vi "Limelight_Differential.vi"() -> (0 "DriveCommand":dbl(knob)=-0.0 scale=-1.0..1.0, 1 "SteerCommand":dbl(knob)=nan scale=-1.0..1.0, 3 "TargetValid":bool)   [LabVIEW 2020]
uses:
  Robot Global Data.vi
panel:
  out "Copy of DriveCommand":dbl format="%_6g"
  out "Limelight tv":dbl
  out "Limelight ta":dbl
  out "Limelight tx":dbl
  out "MaxDrive":dbl(slide)=0.6824817518248175 min=0.0 max=1.0 step=0.01 scale=0.0..1.0
  out "DriveK":dbl(slide)=0.26277372262773724 min=0.0 max=1.0 step=0.05 scale=0.0..1.0
  out "Limelight Goal Area":dbl(slide)=14.872262773722628 min=0.1 max=25.0 step=0.25 scale=0.0..25.0
  out "AimDeadband":dbl min=0.0 max=10.0 step=0.25
  out "MinSteerCommand":dbl(slide)=0.2717391304347826 min=0.0 max=0.5 step=0.05 scale=0.0..0.5
  out "SteeringK":dbl(slide)=0.025362318840579712 min=0.0 max=0.25 step=0.01 scale=0.0..0.25
  # "// These numbers must be tuned for your Robot!  Be careful!\n\n final double STEER_K = 0.03;                    \n// how hard to turn toward the target\n\n\n\n\n \n\nfinal double DESIRED_TARGET_AREA = 13.0;        \n// Area of the target when the robot reaches the wall\n\n\n\nfinal double DRIVE_K = 0.26;                   \n // how hard to drive fwd toward the target\n\n \n \nfinal double MAX_DRIVE = 0.7;                   \n// Simple speed limit so we don't drive too fast"
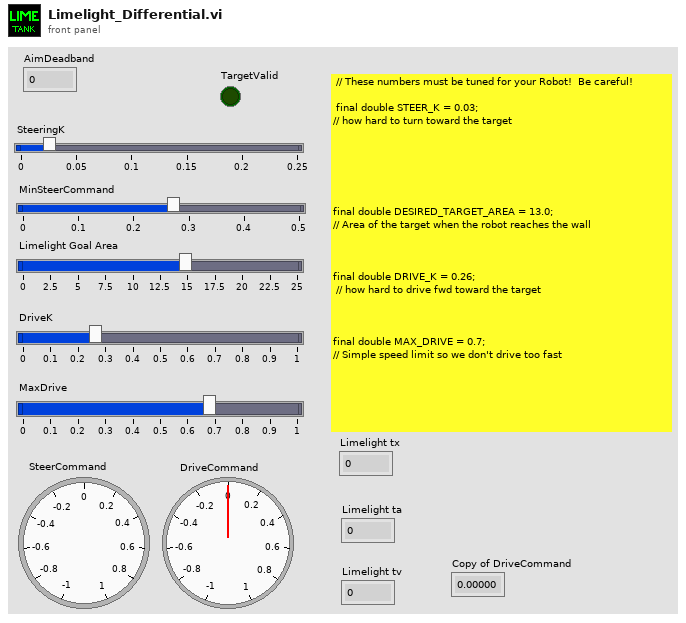
[diagram p1: front panel]
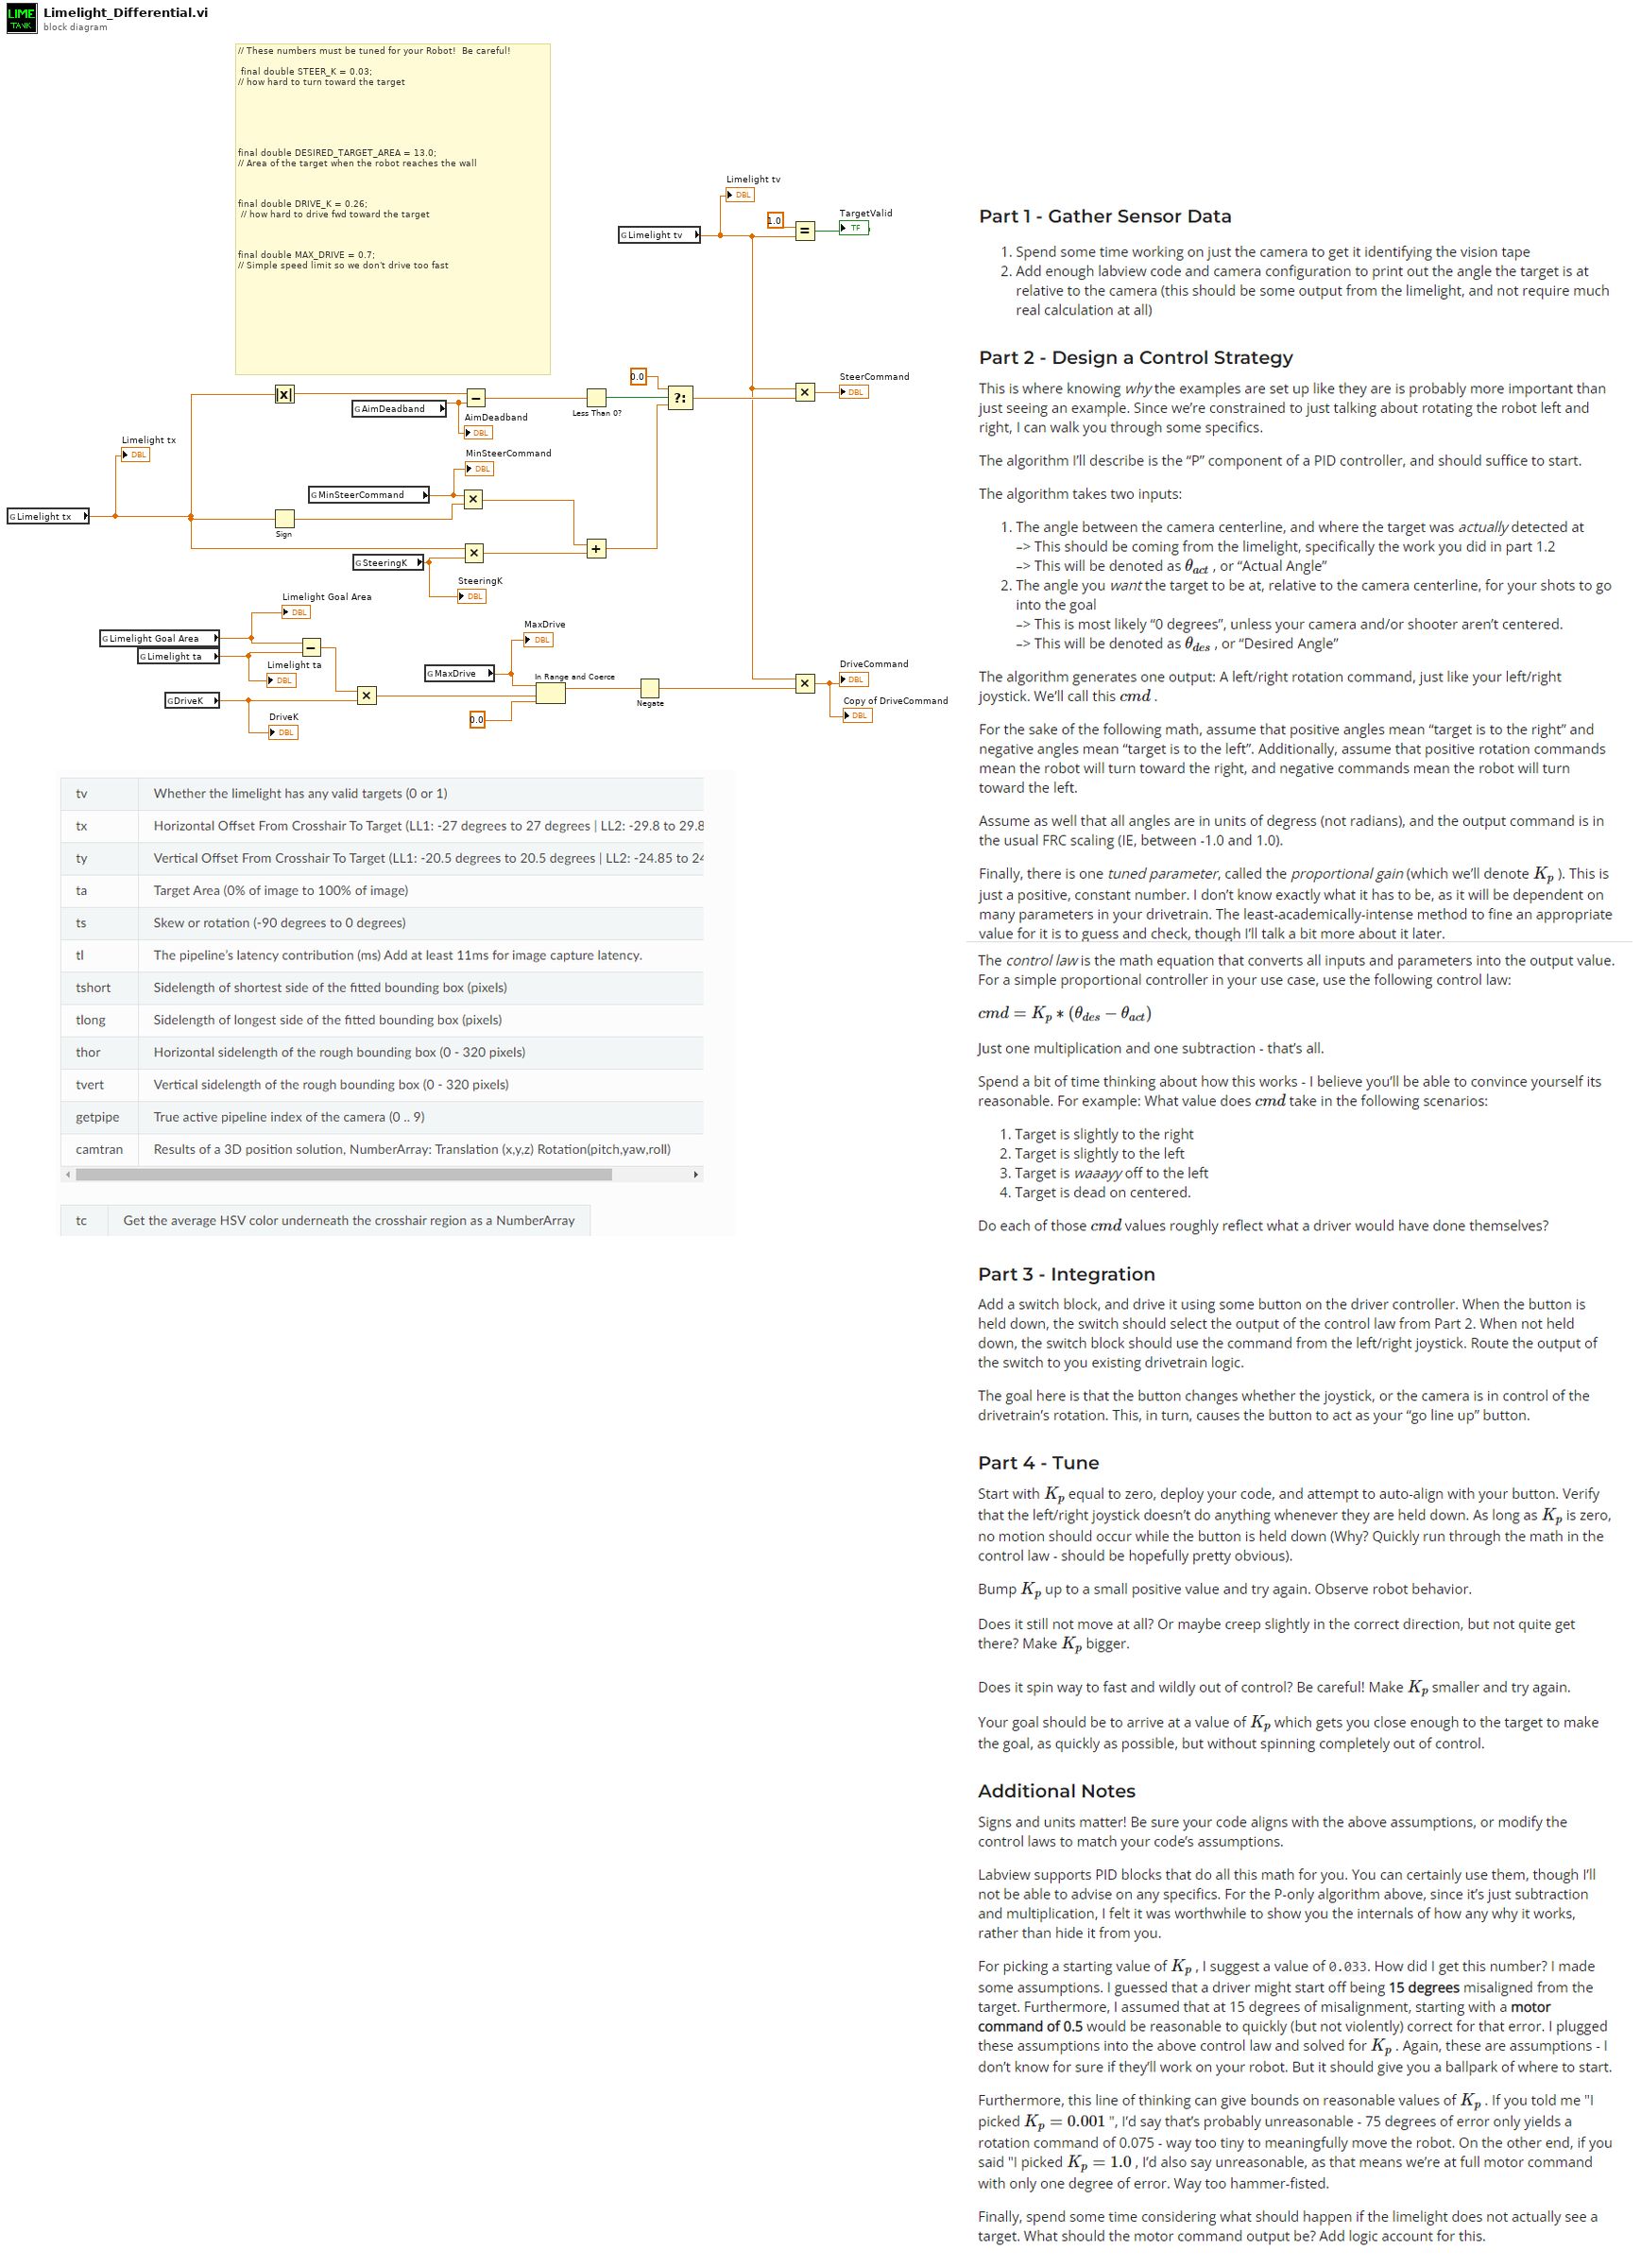
[diagram p0: block diagram]
diagram:
  # "// These numbers must be tuned for your Robot!  Be careful!\n\n final double STEER_K = 0.03;                    \n// how hard to turn toward the target\n\n\n\n\n \n\nfinal double DESIRED_TARGET_AREA = 13.0;        \n// Area of the target when the robot reaches the wall\n\n\n\nfinal double DRIVE_K = 0.26;                   \n // how hard to drive fwd toward the target\n\n \n \nfinal double MAX_DRIVE = 0.7;                   \n// Simple speed limit so we don't drive too fast"
  n1 = global read "Robot Global Data.vi" "Limelight tx"() -> (w10:dbl)
  "Limelight tx" <- w10
  n2 = global read "Robot Global Data.vi" "Limelight Goal Area"() -> (w2:dbl)
  "Limelight Goal Area" <- w2
  n3 = global read "Robot Global Data.vi" "Limelight ta"() -> (w9:dbl)
  "Limelight ta" <- w9
  n4 = global read "Robot Global Data.vi" "DriveK"() -> (w8:dbl)
  "DriveK" <- w8
  n5 = Absolute Value(x=w10) -> (abs(x)=w24:dbl)
  n6 = Sign(1:w10) -> (0:w19:dbl)
  n7 = Subtract(x=w2, y=w9) -> (x-y=w18:dbl)
  n8 = global read "Robot Global Data.vi" "MinSteerCommand"() -> (w4:dbl)
  "MinSteerCommand" <- w4
  n9 = global read "Robot Global Data.vi" "AimDeadband"() -> (w5:dbl)
  "AimDeadband" <- w5
  n10 = Multiply(x=w18, y=w8) -> (x*y=w17:dbl)
  n11 = global read "Robot Global Data.vi" "SteeringK"() -> (w7:dbl)
  "SteeringK" <- w7
  n12 = global read "Robot Global Data.vi" "MaxDrive"() -> (w6:dbl)
  "MaxDrive" <- w6
  n13 = Multiply(x=w4, y=w19) -> (x*y=w23:dbl)
  n14 = Multiply(x=w10, y=w7) -> (x*y=w22:dbl)
  n15 = Subtract(x=w24, y=w5) -> (x-y=w25:dbl)
  n16 = In Range and Coerce(upper limit=w6, x=w17, lower limit=0.0) -> (coerced(x)=w15:dbl)  [unwired: 1 out]
  n17 = Less Than 0?(x=w25) -> (x < 0?=w26:bool)
  n18 = Add(x=w23, y=w22) -> (x+y=w13:dbl)
  n19 = global read "Robot Global Data.vi" "Limelight tv"() -> (w3:dbl)
  "Limelight tv" <- w3
  n20 = Negate(x=w15) -> (-x=w14:dbl)
  n21 = Select(t=0.0, s=w26, f=w13) -> (s? t:f=w21:dbl)
  n22 = Equal?(x=1.0, y=w3) -> (x = y?=→"TargetValid":bool)
  n23 = Multiply(x=w3, y=w21) -> (x*y=→"SteerCommand":dbl)
  n24 = Multiply(x=w3, y=w14) -> (x*y=→"DriveCommand" →"Copy of DriveCommand":dbl)
